vi "RungeKutta.vi"(7 "Oszi-Channel (1)":T1=1.0, 8 "error in (no error)":errorcluster, 9 "Messdaten In":dbl[](array[numeric]), 10 "faktor1":dbl=1.0, 11 "VISA Name OZ In (OZ)":refnum<visa-resource-name>="USB0::0x0957::0x179B::MY54313507::INSTR") -> (0 "error out":errorcluster, 1 "B-Array Out":dbl[](array[numeric]), 3 "VISA Name OZ Out":refnum<visa-resource-name>="USB0::0x0957::0x179B::MY54313507::INSTR")   [LabVIEW 2016]
doc: "Durchfuehren des Runge-Kutta-Verfahrens. um das ueber die Spannung auf das B-Array zu schliessen."
uses:
  controls/Oszi_KanalInfo.ctl
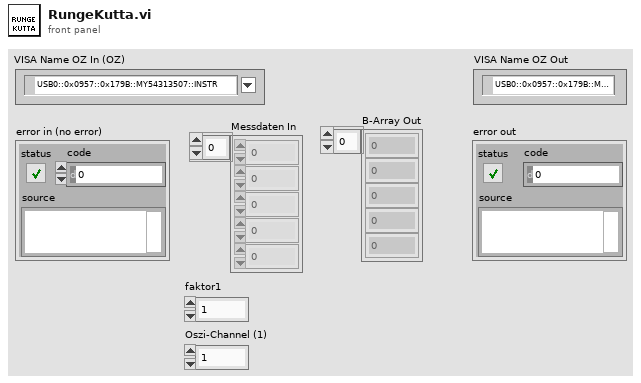
[diagram p1: front panel]
types:
  T1 = typedef "Oszi_KanalInfo.ctl" = dbl
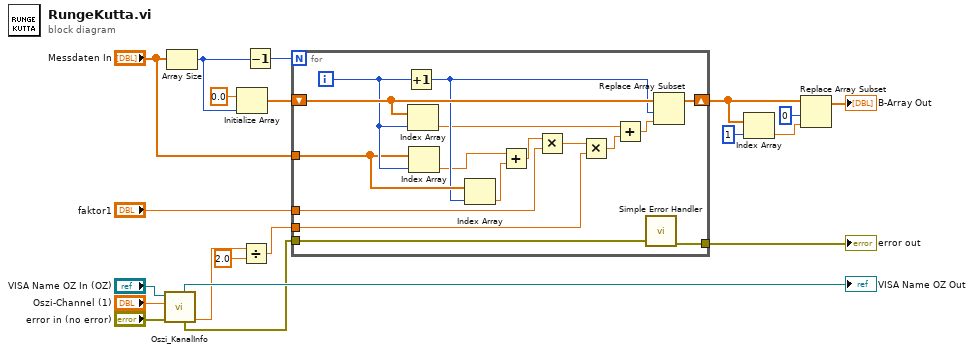
[diagram p0: block diagram]
diagram:
  n1 = call "Oszi_KanalInfo.vi"("Error In (No Error)"="error in (no error)", "Oszi-Channel (1)"="Oszi-Channel (1)", "VISA Name OZ In (OZ)"="VISA Name OZ In (OZ)") -> ("XINcrement"=w15:dbl, "Error Out"=w10:errorcluster, "VISA Name OZ Out"=→"VISA Name OZ Out":refnum<visa-resource-name>)  [unwired: 3 in, 3 out]
  n2 = Array Size(array="Messdaten In") -> (size(s)=w6:i32)
  n3 = Initialize Array(0.0 ("element"), w6) -> (w8:dbl[])
  n4 = Divide(x=w15, y=2.0) -> (x/y=w13:dbl)
  n5 = Decrement(x=w6) -> (x-1=w16:i32)
  n6 = for {
    N: w16 -> [_]
    tunnel: "Messdaten In" -> [w32]
    tunnel: w13 -> [w21]
    shift-right: [w36] -> w3
    shift-left: w8 -> [w35]
    tunnel: "faktor1" -> [w23]
    tunnel: w10 -> [w26]
    tunnel: [w25] -> w9
    i -> [w34]
    n7 = Increment(x=w34) -> (x+1=w31:i32)
    n8 = Index Array(array=w35, index=w34) -> (element=w29:dbl)
    n9 = Index Array(array=w32, index=w34) -> (element=w27:dbl)
    n10 = Index Array(array=w32, index=w31) -> (element=w33:dbl)
    n11 = Add(x=w27, y=w33) -> (x+y=w24:dbl)
    n12 = Multiply(x=w24, y=w23) -> (x*y=w22:dbl)
    n13 = Multiply(x=w22, y=w21) -> (x*y=w30:dbl)
    n14 = Add(x=w29, y=w30) -> (x+y=w28:dbl)
    n15 = call <vilib>:"Simple Error Handler.vi"("error in (no error)"=w26) -> ("error out"=w25:errorcluster)  [unwired: 4 in, 4 out]
    n16 = Replace Array Subset(array=w35, new element=w28, index=w31) -> (w36:dbl[])
  }
  "error out" <- w9
  n17 = Index Array(array=w3, index=1 ("Index")) -> (element=w1:dbl)
  n18 = Replace Array Subset(array=w3, new element=w1, index=0 ("Index")) -> (→"B-Array Out":dbl[])
